vi "WriteMemory.vi"(1 "Value":i32, 2 "Address":i32, 3 "Board":T1(ring)=enum."TIMING_BOARD", 4 "Type":enum16{"X", "Y", "P", "R", "D"}(ring)) -> (0 "Error":bool)   [LabVIEW 2014]
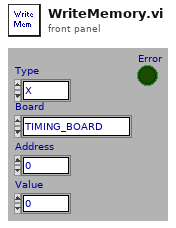
[diagram p1: front panel]
types:
  T1 = enum32{"not used", "PCI_BOARD", "TIMING_BOARD", "UTILITY_BOARD"}
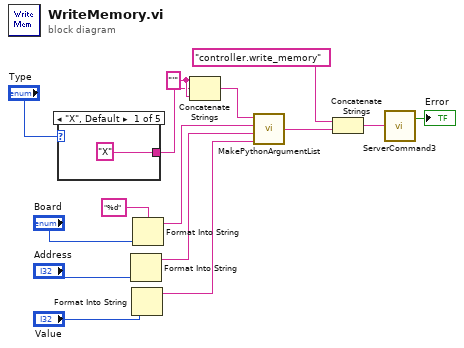
[diagram p0: block diagram]
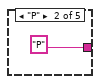
[diagram p2: hidden frame]
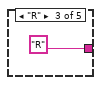
[diagram p3: hidden frame]
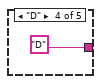
[diagram p4: hidden frame]
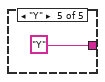
[diagram p5: hidden frame]
diagram:
  w3 = "'" ("string")
  n1 = case shown="\"X\", Default" "Type" {
    tunnel: ["X" "P" "R" "D" "Y"] -> w1
    frame "X", Default {
    }
    frame "P" {
    }
    frame "R" {
    }
    frame "D" {
    }
    frame "Y" {
    }
  }
  n2 = Format Into String("Address") -> (resulting string=w6:string)  [unwired: 3 in, 1 out]
  n3 = Format Into String("Value") -> (resulting string=w5:string)  [unwired: 3 in, 1 out]
  n4 = Format Into String(format string="%d" ("Format String"), "Board") -> (resulting string=w7:string)  [unwired: 2 in, 1 out]
  n5 = Concatenate Strings(w3, w1, w3) -> (w2:string)
  n6 = call "MakePythonArgumentList.vi"("Arg 4"=w5, "Arg 3"=w6, "Arg 2"=w7, "Arg 1"=w2) -> ("Args Out"=w4:string)  [unwired: 2 in]
  n7 = Concatenate Strings("controller.write_memory" ("string"), w4) -> (w8:string)
  n8 = call "ServerCommand3.vi"("Command"=w8) -> ("Error"=→"Error":bool)  [unwired: 1 out]
